vi "ImageTester.vi"() -> ()   [LabVIEW 2017]
panel:
  out "dt(ms)":dbl
  out "PostTime":timestamp
  out "PrevTime":timestamp
  out "ScaleAngleDegrees":dbl
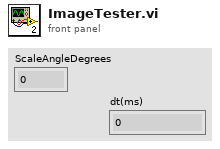
[diagram p1: front panel]
types:
  T1 = typedef "Image Type" = u32
  T2 = typedef "IMAQ Image.ctl" = refnum<image>
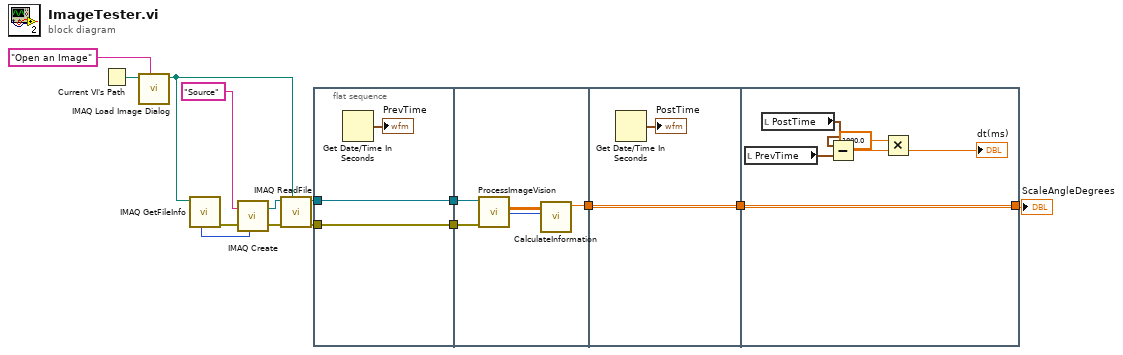
[diagram p0: block diagram]
diagram:
  n1 = Current VI's Path() -> (path=w15:path)
  n2 = call "IMAQ Load Image Dialog"("Prompt"="Open an Image", "Start Path"=w15) -> ("Path"=w10:path)  [unwired: 5 in, 4 out]
  n3 = call "IMAQ GetFileInfo"("File Path"=w10) -> ("error out"=w7:errorcluster, "Image Type"=w12:T1)  [unwired: 1 in, 8 out]
  n4 = call "IMAQ Create"("Image Name"="Source", "Image Type"=w12, "error in (no error)"=w7) -> ("New Image"=w11:T2, "error out"=w6:errorcluster)  [unwired: 1 in, 1 out]
  n5 = call "IMAQ ReadFile"("File Path"=w10, "error in (no error)"=w6, "Image"=w11) -> ("error out"=w8:errorcluster, "Image Out"=w9:T2)  [unwired: 2 in, 5 out]
  n6 = flat-sequence {
    tunnel: w8 -> [w17]
    tunnel: w9 -> [w18]
    tunnel: [w18] -> w3
    tunnel: [w17] -> w2
    tunnel: [w19] -> w4
    tunnel: w3 -> [w23]
    tunnel: w2 -> [w22]
    tunnel: w4 -> [w25]
    tunnel: [w25] -> w1
    tunnel: [w31] -> w5
    tunnel: w1 -> [w31]
    frame #0 {
      n7 = Get Date/Time In Seconds() -> (seconds since 1Jan1904=→"PrevTime":timestamp)
    }
    frame #1 {
      n8 = call "ProcessImageVision.vi"("error in"=w22, "Image In"=w23) -> ("Number of Particles (Particle Analysis 1)"=w20:i32, "Particle Measurements (Pixels) (Particle Analysis 1)"=w21:dbl[][])  [unwired: 3 in, 2 out]
      n9 = call "CalculateInformation.vi"("Number of Particles"=w20, "Particle Measurements"=w21) -> ("ScaleAngleDegrees"=w19:dbl)  [unwired: 9 in]
    }
    frame #2 {
      n10 = Get Date/Time In Seconds() -> (seconds since 1Jan1904=→"PostTime":timestamp)
    }
    frame #3 {
      n11 = local read "PrevTime"() -> (w29:timestamp)
      n12 = local read "PostTime"() -> (w30:timestamp)
      n13 = Subtract(x=w30, y=w29) -> (x-y=w28:dbl)
      n14 = Multiply(x=1000.0, y=w28) -> (x*y=→"dt(ms)":dbl)
    }
  }
  "ScaleAngleDegrees" <- w5
